vi "usb write reg data.vi"(10 "write_data":u8[](array[numeric])=[0, 0], 11 "addr":u8[](array[numeric])=[0, 0]) -> (1 "function return":bool, 2 "write_data out":u8[](array[numeric]), 3 "addr out":u8[](array[numeric]))   [LabVIEW 2018, in "Dll1_x64_191014_0.lvlib"]
doc: "__declspec(dllexport) bool usb_write_reg_data(char addr[2], unsigned char write_data[2]);"
uses:
  Dll1_x64_191014_0.lvlib
  Dll1.dll
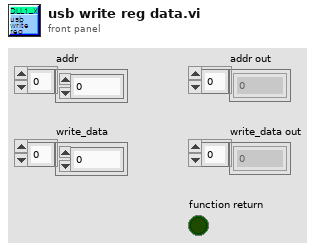
[diagram p1: front panel]
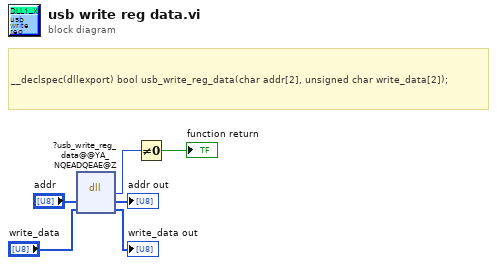
[diagram p0: block diagram]
diagram:
  # "__declspec(dllexport) bool usb_write_reg_data(char addr[2], unsigned char write_data[2]);"
  n1 = dll-call lib="PTH2zabs CUsersLenovoDesktopDHCC실험2#lux image capture_0.9.1.1_Temporaryuser.libDll1_x64_191014_0Dll1.*" fn="?usb_write_reg_data@@YA_NQEADQEAE@Z"("addr"="addr", "write_data"="write_data") -> (w5:u8, "addr"=→"addr out":u8[], "write_data"=→"write_data out":u8[])  [unwired: 3 in, 2 out]
  n2 = Not Equal To 0?(x=w5) -> (x != 0?=→"function return":bool)
